vi "_reorder tool entries.vi"(11 "Path Control":path[](array[path])) -> (3 "After":string[](array[string]))   [LabVIEW 2017, in "CSM DebugTool Dialog.lvlib"]
uses:
  CSM DebugTool Dialog.lvlib
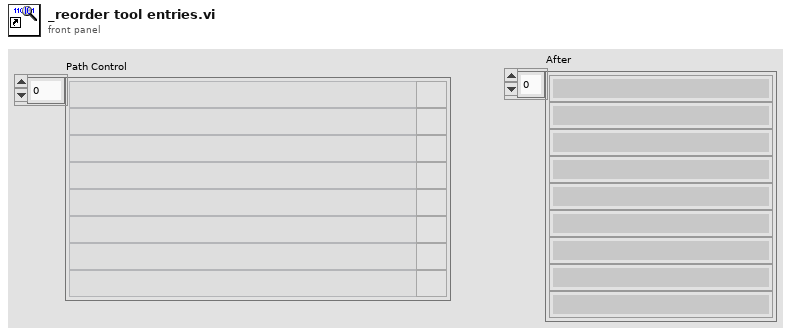
[diagram p1: front panel]
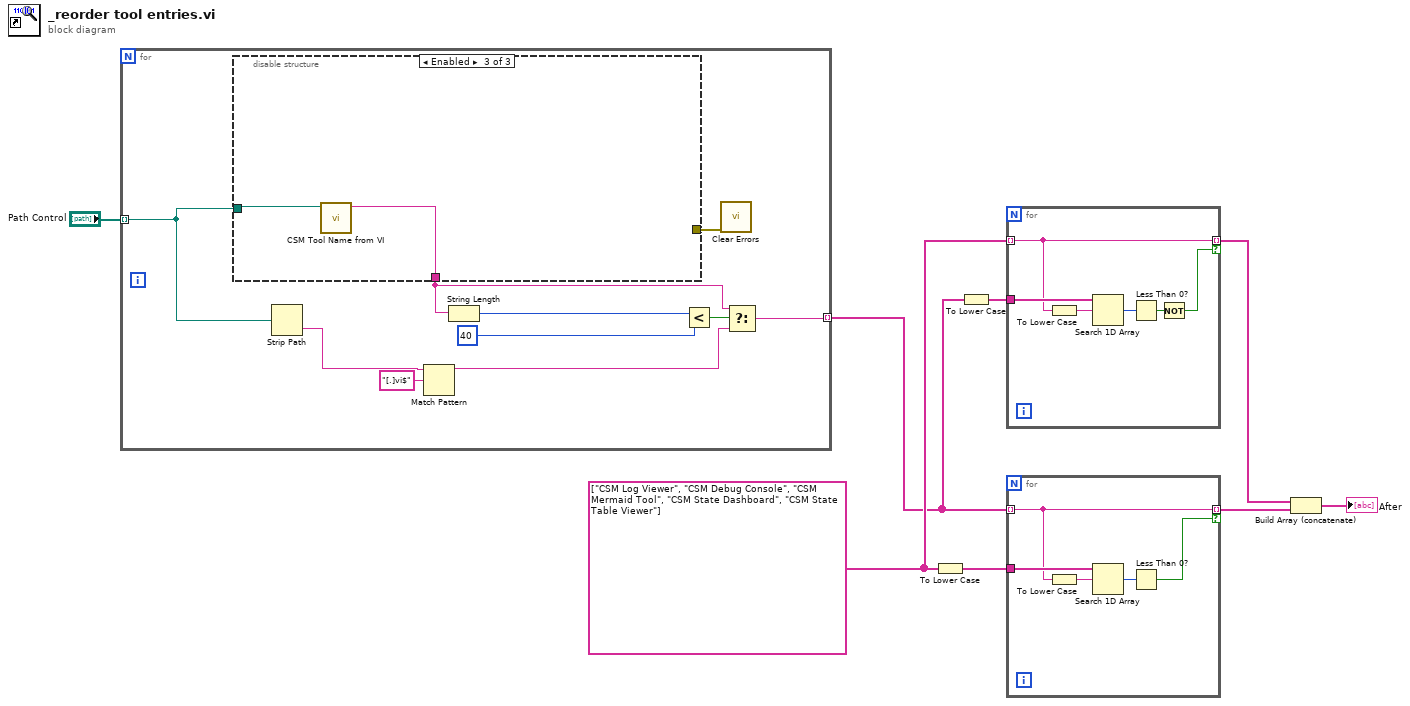
[diagram p0: block diagram]
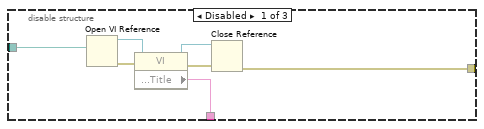
[diagram p2: hidden frame]
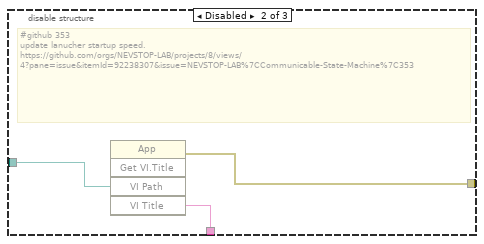
[diagram p3: hidden frame]
diagram:
  w5 = string[] ["CSM Log Viewer", "CSM Debug Console", "CSM Mermaid Tool", "CSM State Dashboard", "CSM State Table Viewer"] ("Before 2")
  n1 = for {
    tunnel: "Path Control" -> [w17] mode=indexing
    tunnel: [w11] -> w1 mode=indexing
    n2 = disable-structure shown="Enabled" {
      disable-tunnel: [w21 w26 _] -> w18
      disable-tunnel: w17 -> [w20 w28 w30]
      disable-tunnel: [w19 w27 w29] -> w15
      frame Disabled {
        n3 = Open VI Reference(vi path=w20) -> (vi reference=w25:refnum<vi>, error out=w24:errorcluster)  [unwired: 5 in]
        n4 = property class="VI"(reference=w25, error in=w24) -> (reference out=w22:refnum<vi>, error out=w23:errorcluster, "Front Panel.Title"=w19:string)
        n5 = Close Reference(reference=w22, error in (no error)=w23) -> (error out=w21:errorcluster)
      }
      frame Disabled {
        # "#github 353\nupdate lanucher startup speed.\nhttps://github.com/orgs/NEVSTOP-LAB/projects/8/views/4?pane=issue&itemId=92238307&issue=NEVSTOP-LAB%7CCommunicable-State-Machine%7C353"
        n6 = invoke class="App" method="Get VI.Title"("VI Path"=w28) -> (error out=w26:errorcluster, "VI Title"=w27:string)  [unwired: 4 in, 3 out]
      }
      frame Enabled {
        n7 = call "CSM Tool Name from VI.vi"("VI Path"=w30) -> ("ToolName"=w29:string)  [unwired: 10 in]
      }
    }
    n8 = Strip Path(path=w17) -> (name=w14:string)  [unwired: 1 out]
    n9 = Match Pattern(string=w14, regular expression="[.]vi$") -> (before substring=w12:string)  [unwired: 1 in, 3 out]
    n10 = String Length(string=w15) -> (length=w10:i32)
    n11 = Less?(x=w10, y=40) -> (x < y?=w16:bool)
    n12 = call <vilib>:"Clear Errors.vi"("error in (no error)"=w18) -> ()  [unwired: 5 in, 2 out]
    n13 = Select(t=w15, s=w16, f=w12) -> (s? t:f=w11:string)
  }
  n14 = To Lower Case(string=w5) -> (all lower case string=w7:string[])
  n15 = To Lower Case(string=w1) -> (all lower case string=w3:string[])
  n16 = for {
    tunnel: [w35] -> w4 mode=indexing if=w31
    tunnel: w5 -> [w35] mode=indexing
    tunnel: w3 -> [w36]
    n17 = To Lower Case(string=w35) -> (all lower case string=w34:string)
    n18 = Search 1D Array(1D array=w36, element=w34) -> (index of element=w33:i32)  [unwired: 1 in]
    n19 = Less Than 0?(x=w33) -> (x < 0?=w32:bool)
    n20 = Not(x=w32) -> (.not. x?=w31:bool)
  }
  n21 = for {
    tunnel: [w40] -> w8 mode=indexing if=w37
    tunnel: w1 -> [w40] mode=indexing
    tunnel: w7 -> [w41]
    n22 = To Lower Case(string=w40) -> (all lower case string=w39:string)
    n23 = Search 1D Array(1D array=w41, element=w39) -> (index of element=w38:i32)  [unwired: 1 in]
    n24 = Less Than 0?(x=w38) -> (x < 0?=w37:bool)
  }
  n25 = Build Array (concatenate)(w4, w8) -> (→"After":string[])
